vi "Read Data Matrix Code.vi"() -> ()   [LabVIEW 2014]
doc: "This example illustrates how to use the Read Data Matrix Barcode VI. There are several types of DataMatrix barcodes that are supported including ECC 000-140, ECC 200 as well as various cell shapes and barcode shapes."
uses:
  <vilib>/vision/Instrument.llb/Data Matrix Search Options.ctl
  <vilib>/vision/Instrument.llb/Demodulation Mode.ctl
  <vilib>/vision/Instrument.llb/Cell Sample Size.ctl
  <vilib>/vision/Instrument.llb/Cell Filter Mode.ctl
  <vilib>/vision/Instrument.llb/Data Matrix Size Options.ctl
  <vilib>/vision/Instrument.llb/Data Matrix Description Options.ctl
  <vilib>/vision/Instrument.llb/ECC Type.ctl
  <vilib>/vision/Instrument.llb/Data Matrix Polarity.ctl
  <vilib>/vision/Instrument.llb/Cell Fill Percentage.ctl
  <vilib>/vision/Instrument.llb/Data Matrix Mirror.ctl
  <vilib>/vision/NI_Vision_Development_Module.lvlib
panel:
  out "Read Time (ms)":dbl format="%.2f"
  out "Data":string
  out "Image":T1(plugin-control)
  # "Overview: Demonstrate the reading of Data Matrix barcode\nRequirements: Vision Development Module.\nInstructions: Run the VI."
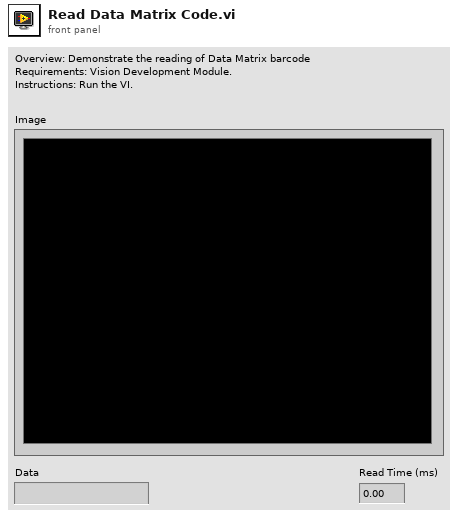
[diagram p1: front panel]
types:
  T1 = typedef "IMAQ Image.ctl" = refnum<image>
  T2 = typedef "Data Matrix Description Options.ctl" = cluster{"Aspect Ratio":sgl, "Rows":u32, "Columns":u32, "Rectangle":bool, "ECC":T3, "Barcode Polarity":T4, "Cell Fill Percentage":T5, "Minimum Border Integrity %":sgl, "Mirror Mode":T6}
  T3 = typedef "ECC Type.ctl" = i32
  T4 = typedef "Data Matrix Polarity.ctl" = i32
  T5 = typedef "Cell Fill Percentage.ctl" = i32
  T6 = typedef "Data Matrix Mirror.ctl" = i32
  T7 = typedef "Data Matrix Size Options.ctl" = cluster{"Data Matrix Size":cluster{"Minimum Size":u32, "Maximum Size":u32}, "Quiet Zone Width":u32}
  T8 = typedef "Data Matrix Search Options.ctl" = cluster{"Rotation Mode":enum32{"Unlimited", "0 Degrees", "90 Degrees", "180 Degrees", "270 Degrees"}, "Skip Location?":bool, "Edge Threshold":u32, "Demodulation Mode":T9, "Cell Sample Size":T10, "Cell Filter Mode":T11, "Skew Degrees Allowed":u32, "Maximum Iterations":u32, "Initial Search Vector Width":u32}
  T9 = typedef "Demodulation Mode.ctl" = i32
  T10 = typedef "Cell Sample Size.ctl" = i32
  T11 = typedef "Cell Filter Mode.ctl" = i32
  T12 = typedef "Data Matrix Report.ctl" = cluster{"Found?":bool, "Binary?":bool, "Data":string, "Bounding Box":cluster{"x":sgl, "y":sgl}[], "Errors Corrected":u32, "Erasures Corrected":u32, "Aspect Ratio":sgl, "Rows":u32, "Columns":u32, "ECC":T3, "Barcode Polarity":T4, "Cell Fill Percentage":T5, "Border Integrity":sgl, "Mirrored?":bool, "Minimum Edge Strength":u32, "Demodulation Mode":T9, "Cell Sample Size":T10, "Cell Filter Mode":T11, "Iterations":u32}
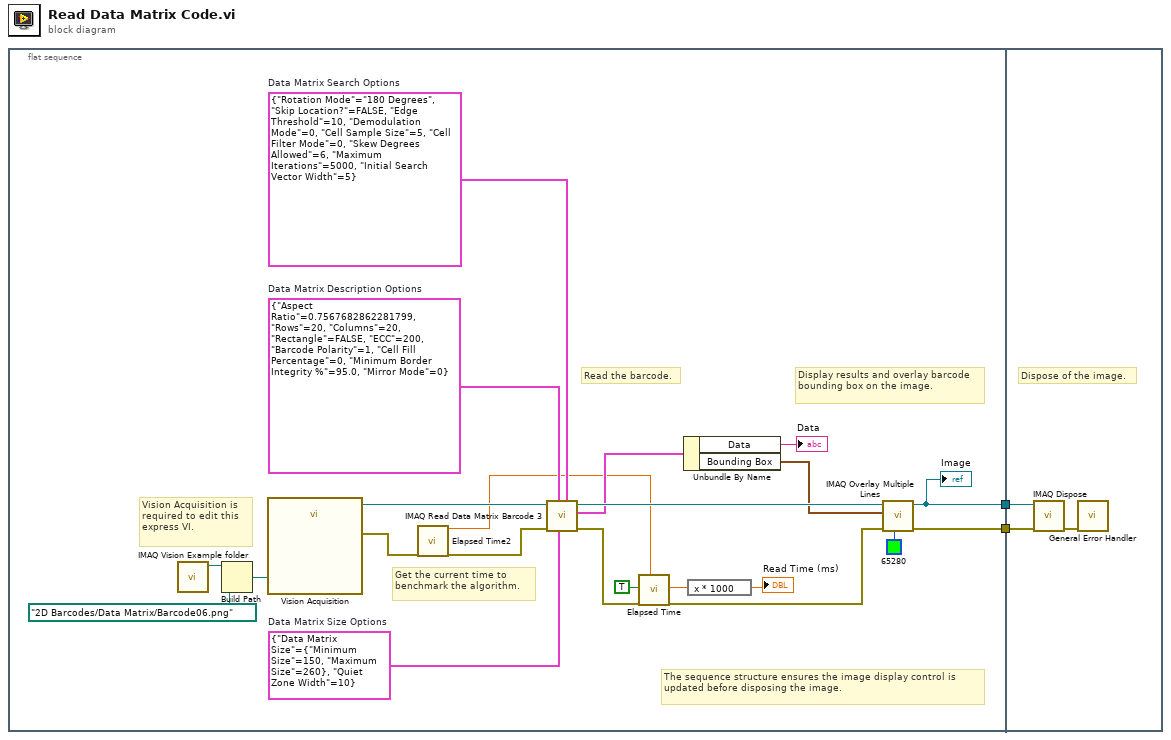
[diagram p0: block diagram]
diagram:
  n1 = flat-sequence {
    tunnel: [w24] -> w2
    tunnel: [w23] -> w1
    tunnel: w2 -> [w26]
    tunnel: w1 -> [w25]
    frame #0 {
      w9 = T2 {"Aspect Ratio"=0.7567683, "Rows"=20, "Columns"=20, "Rectangle"=FALSE, "ECC"=200, "Barcode Polarity"=1, "Cell Fill Percentage"=0, "Minimum Border Integrity %"=95.0, "Mirror Mode"=0}  # Data Matrix Description Options
      w8 = T7 {"Data Matrix Size"={"Minimum Size"=150, "Maximum Size"=260}, "Quiet Zone Width"=10}  # Data Matrix Size Options
      w10 = T8 {"Rotation Mode"=enum."180 Degrees", "Skip Location?"=FALSE, "Edge Threshold"=10, "Demodulation Mode"=0, "Cell Sample Size"=5, "Cell Filter Mode"=0, "Skew Degrees Allowed"=6, "Maximum Iterations"=5000, "Initial Search Vector Width"=5}  # Data Matrix Search Options
      # "The sequence structure ensures the image display control is updated before disposing the image."
      # "Vision Acquisition is required to edit this express VI."
      # "Read the barcode."
      # "Get the current time to benchmark the algorithm."
      # "Display results and overlay barcode bounding box on the image."
      n2 = call "IMAQ Vision Example folder.vi"() -> ("Example Image Path"=w22:path)  [unwired: 11 in]
      n3 = Build Path(base path=w22, name or relative path=path "2D Barcodes/Data Matrix/Barcode06.png" ("path out")) -> (appended path=w11:path)
      n4 = call "Vision Acquisition"("Image Path"=w11) -> ("Image Out"=w19:T1, "error out"=w14:errorcluster)  [unwired: 25 in]
      n5 = call "Elapsed Time2"("error in (no error)"=w14) -> ("Present (s)"=w4:dbl, "error out"=w13:errorcluster)  [unwired: 11 in, 6 out]
      n6 = call "IMAQ Read Data Matrix Barcode 3"("Data Matrix Search Options"=w10, "Data Matrix Size Options"=w8, "Data Matrix Description Options"=w9, "error in (no error)"=w13, "Image"=w19) -> ("error out"=w6:errorcluster, "Data Matrix Report"=w15:T12, "Image (duplicate)"=w17:T1)  [unwired: 3 in, 1 out]
      n7 = call "Elapsed Time"("Reset"=TRUE, "error in (no error)"=w6, "Set Start Time (s)"=w4) -> ("Elapsed Time (s)"=w20:dbl, "error out"=w5:errorcluster)  [unwired: 9 in, 6 out]
      n8 = Unbundle By Name(w15) -> ("Data"=→"Data":string, "Bounding Box"=w16:cluster{"x":sgl, "y":sgl}[])
      n9 = expression code="x * 1000"(w20) -> (→"Read Time (ms)":dbl)
      n10 = call "IMAQ Overlay Multiple Lines"("Color"=u32 65280, "error in (no error)"=w5, "Line End Points"=w16, "Image"=w17) -> ("error out"=w23:errorcluster, "Image Out"=w24:T1)  [unwired: 6 in]
      "Image" <- w24
    }
    frame #1 {
      # "Dispose of the image."
      n11 = call "IMAQ Dispose"("Image"=w26, "error in (no error)"=w25) -> ("error out"=w27:errorcluster)  [unwired: 4 in]
      n12 = call <vilib>:"General Error Handler.vi"("error in (no error)"=w27) -> ()  [unwired: 10 in, 5 out]
    }
  }
